vi "FormatFunctionCall.vi"(1 "parameters":string[](array[string]), 2 "function":string) -> (0 "python object":string)   [LabVIEW 2014, in "Python Functions.lvlib"]
uses:
  Python Functions.lvlib
  ListTypesTD.ctl
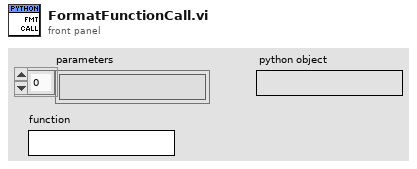
[diagram p1: front panel]
types:
  T1 = typedef "Python Functions.lvlib/ListTypesTD.ctl" = enum16{"list", "tuple", "parameter list", "output list"}
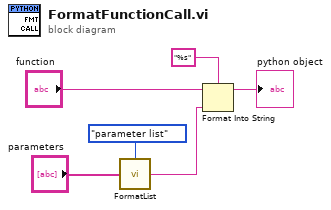
[diagram p0: block diagram]
diagram:
  n1 = call "FormatList.vi"("values"="parameters", "type"=ListTypesTD."parameter list") -> ("python object"=w3:string)
  n2 = Format Into String(format string="%s", initial string="function", w3) -> (resulting string=→"python object":string)  [unwired: 1 in, 1 out]
